vi "Update.vi"(8 "error in (no error)":errorcluster, 10 "Message in":refnum<class "UpdateMessage.lvclass">, 11 "StageSPIM in":refnum<class "StageSPIM.lvclass">) -> (0 "error out":errorcluster, 3 "StageSPIM out":refnum<class "StageSPIM.lvclass">)   [LabVIEW 2012, in "StageSPIM.lvclass"]
doc: "The update method processes the command 'update'. \n\nThe command 'update' is used for receiving new values to be set to the private data of the class. This could be seen as a public set method for setting new parameters to the private class data."
uses:
  StageSPIM.lvclass
  <vilib>/Distrio/Murmex/Murmex/Murmex.lvclass
  <vilib>/Distrio/Murmex/UpdateMessage/UpdateMessage.lvclass
panel:
  # "This method is called when the UPDATE\ntrigger is sent. \n\nOverride this method when your component needs to\nrespond to this trigger. \n\nCall parent for proper implementation"
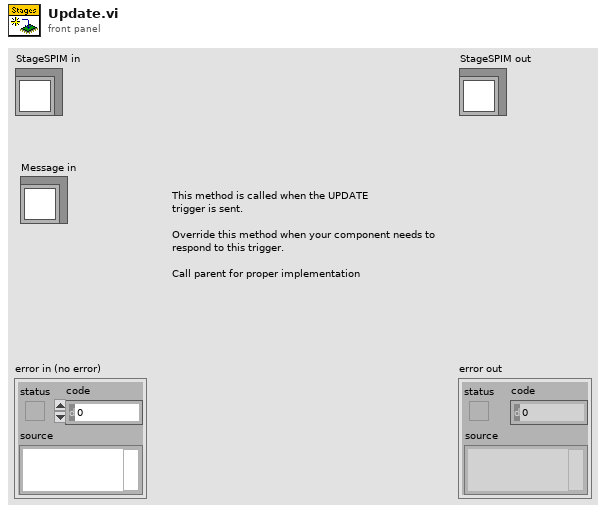
[diagram p1: front panel]
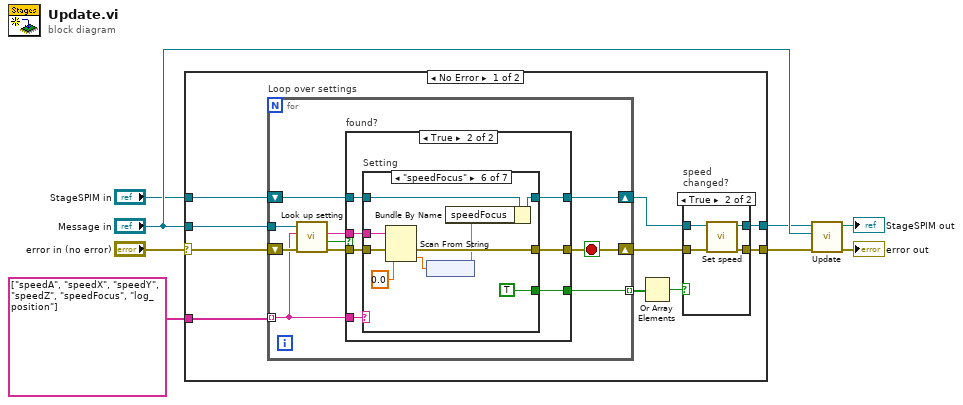
[diagram p0: block diagram]
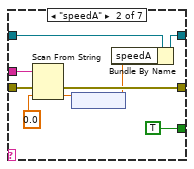
[diagram p5: hidden frame]
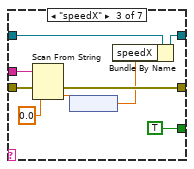
[diagram p6: hidden frame]
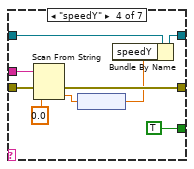
[diagram p7: hidden frame]
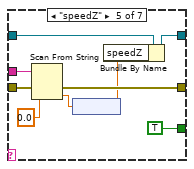
[diagram p8: hidden frame]
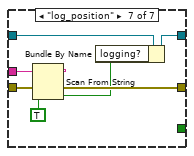
[diagram p9: hidden frame]
diagram:
  n1 = case shown="No Error" "error in (no error)" {
    selector: "error in (no error)" -> [w18 w98]
    tunnel: [w13 w98] -> w5
    tunnel: string[] ["speedA", "speedX", "speedY", "speedZ", "speedFocus", "log_position"] ("key chains") -> [w17 _]
    tunnel: "Message in" -> [w16 _]
    tunnel: "StageSPIM in" -> [w15 w99]
    tunnel: [w11 w99] -> w1
    frame No Error {
      n2 = for "Loop over settings" {
        shift-right: [w26] -> w14
        shift-left: w18 -> [w34]
        tunnel: w17 -> [w28] mode=indexing
        tunnel: w16 -> [w33]
        shift-right: [w27] -> w12
        shift-left: w15 -> [w31]
        tunnel: [w25] -> w10 mode=indexing
        stop <- w26 stop-if-true
        n3 = call <vilib>:"Look up setting.vi"("error in (no error)"=w34, "tag name"=w28, "UpdateMessage in"=w33) -> ("error out"=w29:errorcluster, "found?"=w32:bool, "value"=w30:string)  [unwired: 5 in, 1 out]
        n4 = case "found?" shown="True" w32 {
          tunnel: w31 -> [w36 w41]
          tunnel: w30 -> [_ w42]
          tunnel: w29 -> [w35 w40]
          tunnel: w28 -> [_ w43]
          tunnel: [w36 w39] -> w27
          tunnel: [w35 w38] -> w26
          tunnel: [_ w37] -> w25
          frame False {
          }
          frame True {
            n5 = case "Setting" shown="\"speedFocus\"" w43 {
              tunnel: w42 -> [_ w50 w62 w67 w77 w86 w95]
              tunnel: w41 -> [w45 w52 w61 w71 w80 w89 w93]
              tunnel: w40 -> [w44 w54 w63 w72 w81 w90 w97]
              tunnel: [w45 w51 w60 w70 w79 w88 w92] -> w39
              tunnel: [w44 w53 w59 w68 w78 w87 w96] -> w38
              tunnel: [_ TRUE TRUE TRUE TRUE TRUE _] -> w37
              frame Default {
              }
              frame "speedA" {
                n6 = Scan From String(input string=w50, error in=w54, default 1=0.0 ("Settings_cluster.Power")) -> (error out=w53:errorcluster, output 1=w49:dbl)  [unwired: 2 in, 2 out]
                n7 = node(w49) -> (w48:dbl[unit])
                n8 = Bundle By Name(cluster=w52, "speedA"=w48) -> (w51:refnum<class "StageSPIM.lvclass">)
              }
              frame "speedX" {
                n9 = Scan From String(input string=w62, error in=w63, default 1=0.0 ("Settings_cluster.Power")) -> (error out=w59:errorcluster, output 1=w58:dbl)  [unwired: 2 in, 2 out]
                n10 = node(w58) -> (w57:dbl[unit])
                n11 = Bundle By Name(cluster=w61, "speedX"=w57) -> (w60:refnum<class "StageSPIM.lvclass">)
              }
              frame "speedY" {
                n12 = Scan From String(input string=w67, error in=w72, default 1=0.0 ("Settings_cluster.Power")) -> (error out=w68:errorcluster, output 1=w66:dbl)  [unwired: 2 in, 2 out]
                n13 = node(w66) -> (w65:dbl[unit])
                n14 = Bundle By Name(cluster=w71, "speedY"=w65) -> (w70:refnum<class "StageSPIM.lvclass">)
              }
              frame "speedZ" {
                n15 = Scan From String(input string=w77, error in=w81, default 1=0.0 ("Settings_cluster.Power")) -> (error out=w78:errorcluster, output 1=w76:dbl)  [unwired: 2 in, 2 out]
                n16 = node(w76) -> (w75:dbl[unit])
                n17 = Bundle By Name(cluster=w80, "speedZ"=w75) -> (w79:refnum<class "StageSPIM.lvclass">)
              }
              frame "speedFocus" {
                n18 = Scan From String(input string=w86, error in=w90, default 1=0.0 ("Settings_cluster.Power")) -> (error out=w87:errorcluster, output 1=w85:dbl)  [unwired: 2 in, 2 out]
                n19 = node(w85) -> (w84:dbl[unit])
                n20 = Bundle By Name(cluster=w89, "speedFocus"=w84) -> (w88:refnum<class "StageSPIM.lvclass">)
              }
              frame "log_position" {
                n21 = Scan From String(input string=w95, error in=w97, default 1=TRUE) -> (error out=w96:errorcluster, output 1=w91:bool)  [unwired: 2 in, 2 out]
                n22 = Bundle By Name(cluster=w93, "logging?"=w91) -> (w92:refnum<class "StageSPIM.lvclass">)
              }
            }
          }
        }
      }
      n23 = Or Array Elements(Boolean array=w10) -> (logical OR=w9:bool)
      n24 = case "speed\nchanged?" shown="True" w9 {
        tunnel: w14 -> [w19 w24]
        tunnel: [w19 w23] -> w13
        tunnel: w12 -> [w20 w22]
        tunnel: [w20 w21] -> w11
        frame False {
        }
        frame True {
          n25 = call-dynamic "Set speed.vi"("error in (no error)"=w24, "StageSPIM in"=w22) -> ("error out"=w23:errorcluster, "StageSPIM out"=w21:refnum<class "StageSPIM.lvclass">)  [unwired: 8 in]
        }
      }
    }
    frame Error {
    }
  }
  n26 = call-parent "Update.vi"("error in (no error)"=w5, "Message in"="Message in", "Murmex in"=w1) -> ("error out"=→"error out":errorcluster, "Murmex out"=→"StageSPIM out":refnum<class "StageSPIM.lvclass">)  [unwired: 7 in]
